vi "Q - not nan and gtr than zero - Integer.vi"(10 "Numeric":i32) -> (2 "Boolean":bool=TRUE)   [LabVIEW 2010]
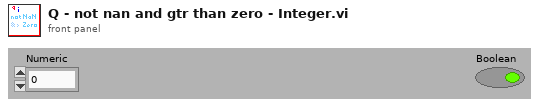
[diagram p1: front panel]
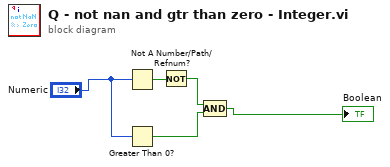
[diagram p0: block diagram]
diagram:
  n1 = Not A Number/Path/Refnum?(number/path/refnum="Numeric") -> (NaN/Path/Refnum?=w5:bool)
  n2 = Greater Than 0?(x="Numeric") -> (x > 0?=w3:bool)
  n3 = Not(x=w5) -> (.not. x?=w2:bool)
  n4 = Compound Arithmetic op=AND(w2, w3) -> (→"Boolean":bool)
